vi "OxITC503 _VISA_ Initialise.vi"(2 "Timeout Value (default 5000)":u32=5000, 3 "error in (no error)":errorcluster, 5 "VISA session":refnum<visa-resource-name>) -> (0 "error out":errorcluster, 1 "VISA session":refnum<visa-resource-name>)   [LabVIEW 2013]
doc: "Initialises the interface of the device, sets the timeout for the communication, the end of message character to CR, and enables Service Request VISA event.\n\nService Request (default) 0x3FFF200B.\n\nNotifies the application that a service request was received from the device or interface associated with the given session. \n\nNote:\n When you receive this event on an instrument session, you must call VISA Read STB to guarantee delivery of future service request events on the given session."
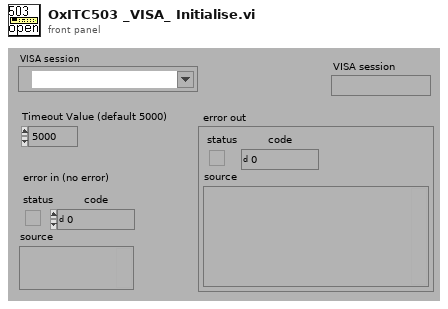
[diagram p1: front panel]
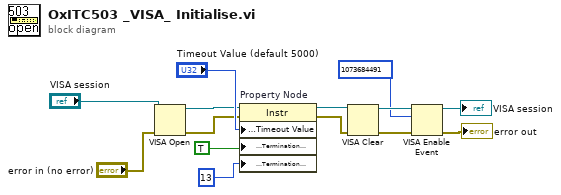
[diagram p0: block diagram]
diagram:
  n1 = VISA Open(error in (no error)="error in (no error)", VISA resource name="VISA session") -> (VISA resource name=w4:refnum<visa-resource-name>, error out=w3:errorcluster)  [unwired: 3 in]
  n2 = property on="Property Node" class="Instr"(reference=w4, error in=w3, "General Settings:Timeout Value"="Timeout Value (default 5000)", "Message Based Settings:Termination Character Enable"=TRUE, "Message Based Settings:Termination Character"=u8 13) -> (reference out=w12:refnum<visa-resource-name>, error out=w11:errorcluster)
  n3 = VISA Clear(VISA resource name=w12, error in (no error)=w11) -> (VISA resource name out=w10:refnum<visa-resource-name>, error out=w8:errorcluster)
  n4 = VISA Enable Event(8:w8, 10:u32 1073684491 ("event type"), 11:w10) -> (0:→"error out":errorcluster, 3:→"VISA session":refnum<visa-resource-name>)  [unwired: 1 in]
